vi "1er_Examen.vi"() -> ()   [LabVIEW 2020]
uses:
  <vilib>/numeric/Random Number (Range) DBL.vi
panel:
  out "Random_Value 2":dbl
  out "Random_Value":dbl
  out "Random":dbl[](array[numeric])
  out "EMA":dbl[](array[numeric])
  in  "stop":bool
  in  "Clean Data \nSave":bool caption="Reset"
  in  "Valor Min.":dbl
  in  "Valor Max.":dbl
  out "Tiempo en límite máx.":i64=10
  out "Histeresis 2":bool
  out "Dentro del Rango.":bool
  out "Histeresis":bool
  out "Waveform Graph":cluster{dbl, dbl, dbl[][]}(graph)
  out "?":bool
  in  "# Datos \nalmacenados":i32=5
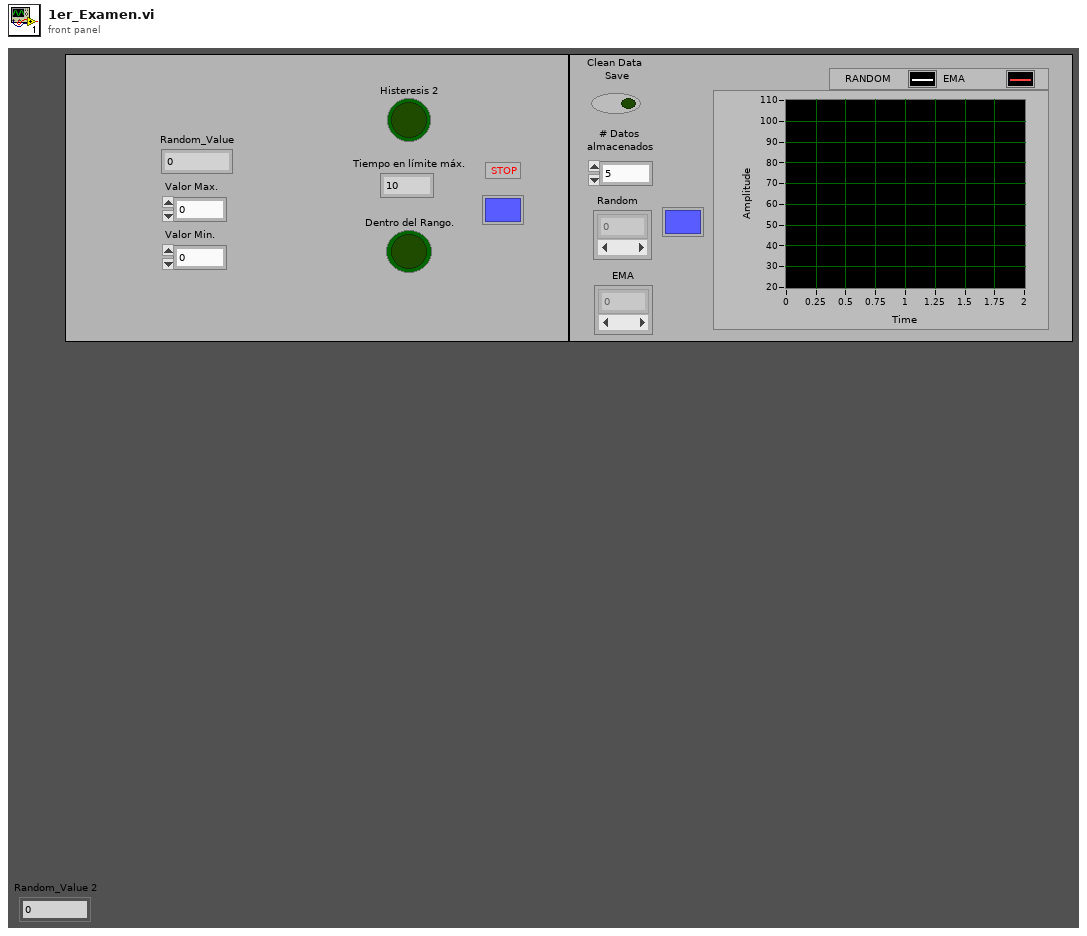
[diagram p1: front panel]
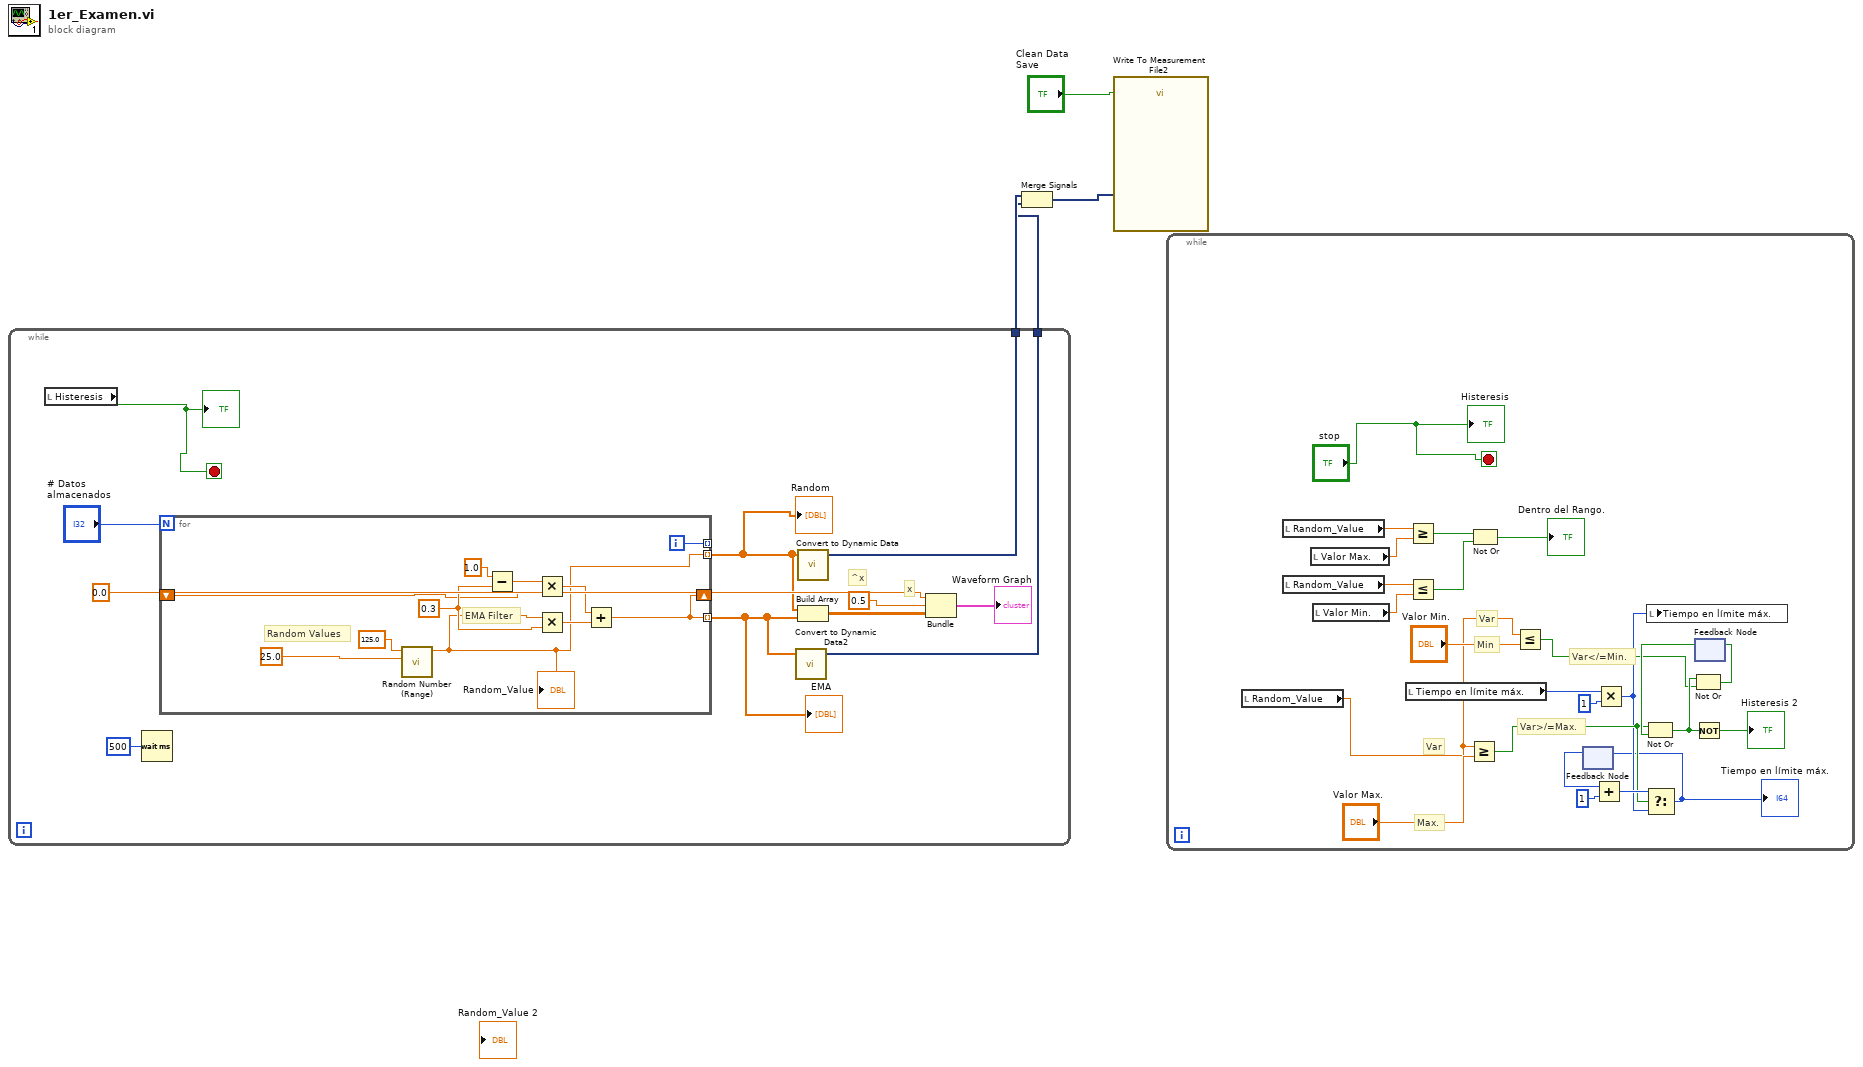
[diagram p0: block diagram]
diagram:
  n1 = while {
    tunnel: [w9] -> w2
    tunnel: [w8] -> w1
    stop <- w5 stop-if-true
    # "^x"
    # "x"
    n2 = local read "Histeresis"() -> (w5:bool)
    "?" <- w5
    n3 = Wait (ms)(milliseconds to wait=u32 500) -> ()  [unwired: 1 out]
    n4 = for {
      N: "# Datos \nalmacenados" -> [_]
      shift-right: [w21] -> _
      shift-left: _ -> [w22]
      tunnel: [w21] -> w7 mode=indexing
      tunnel: [w16] -> w6 mode=indexing
      tunnel: [w17] -> _ mode=indexing
      i -> [w17]
      w24 = 0.3 ("y")
      # "Random Values"
      # "EMA Filter"
      n5 = call-poly <vilib>:"Random Number (Range).vi"("lower bound (0)"=25.0, "upper bound (100)"=125.0) -> ("number"=w16:dbl)  [unwired: 9 in]
      "Random_Value" <- w16
      n6 = Subtract(x=1.0, y=w24) -> (x-y=w26:dbl)
      n7 = Multiply(x=w26, y=w22) -> (x*y=w20:dbl)
      n8 = Multiply(x=w16, y=w24) -> (x*y=w25:dbl)
      n9 = Add(x=w20, y=w25) -> (x+y=w21:dbl)
    }
    "EMA" <- w7
    "Random" <- w6
    n10 = call "Convert to Dynamic Data2"("Array"=w7) -> ("Dynamic Data Type"=w8:dynamicdata)  [unwired: 3 in]
    n11 = call "Convert to Dynamic Data"("Array"=w6) -> ("Dynamic Data Type"=w9:dynamicdata)  [unwired: 3 in]
    n12 = Build Array(w6, w7) -> (w12:dbl[][])
    n13 = Bundle(0.0, 0.5, w12) -> (→"Waveform Graph":cluster{dbl, dbl, dbl[][]})  [unwired: 1 in]
  }
  n14 = Merge Signals(w2, w1) -> (w3:dynamicdata)
  n15 = call "Write To Measurement File2"("Signals"=w3, "Reset"="Clean Data \nSave") -> ()  [unwired: 15 in, 3 out]
  n16 = while {
    stop <- "stop" stop-if-true
    # "Var>/=Max."
    # "Var</=Min."
    # "Var"
    # "Min"
    # "Max."
    # "Var"
    n17 = local read "Random_Value"() -> (w27:dbl)
    n18 = local read "Random_Value"() -> (w37:dbl)
    n19 = local read "Random_Value"() -> (w36:dbl)
    n20 = local read "Valor Max."() -> (w38:dbl)
    n21 = local read "Valor Min."() -> (w35:dbl)
    n22 = local read "Tiempo en límite máx."() -> (w44:i64)
    n23 = Greater Or Equal?(x=w37, y=w38) -> (x >= y?=w33:bool)
    n24 = Less Or Equal?(x=w36, y=w35) -> (x <= y?=w34:bool)
    n25 = Greater Or Equal?(x=w27, y="Valor Max.") -> (x >= y?=w41:bool)
    n26 = Not Or(1:w34, 2:w33) -> (0:→"Dentro del Rango.":bool)
    n27 = Less Or Equal?(x=w27, y="Valor Min.") -> (x <= y?=w40:bool)
    n28 = feedback #1() -> (w31:i64)  [unwired: 1 in]
    n29 = Add(x=w31, y=i64 1) -> (x+y=w45:i64)
    n30 = Multiply(x=w44, y=i64 1 ("f")) -> (x*y=w30:i64)
    n31 = Select(t=w45, s=w41, f=w30) -> (s? t:f=w29:i64)
    "Tiempo en límite máx." <- w29
    n32 = feedback-in #1(w29) -> ()
    n33 = local write "Tiempo en límite máx."(w30) -> ()
    n34 = feedback #2() -> (w50:bool)  [unwired: 1 in]
    n35 = Not Or(1:w50, 2:w41) -> (0:w43:bool)
    n36 = Not Or(1:w40, 2:w43) -> (0:w42:bool)
    n37 = Not(x=w43) -> (.not. x?=→"Histeresis 2":bool)
    n38 = feedback-in #2(w42) -> ()
    "Histeresis" <- "stop"
  }
